vi "cluster2array_for_overlay.vi"(11 "side of clusters":cluster{"Array out":dbl[][]}[](array[cluster])) -> (0 "Left side points":cluster{"X":i32, "Y":i32}[](array[cluster]), 1 "Bottom side points":cluster{"X":i32, "Y":i32}[](array[cluster]), 2 "Right side points":cluster{"X":i32, "Y":i32}[](array[cluster]), 3 "Top side points":cluster{"X":i32, "Y":i32}[](array[cluster]))   [LabVIEW 2017]
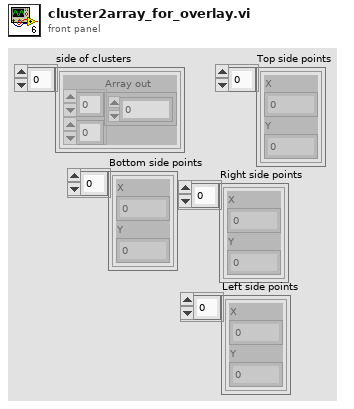
[diagram p1: front panel]
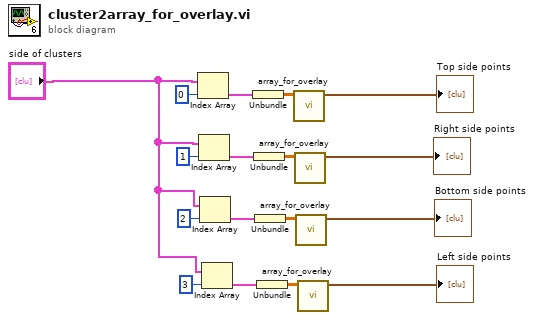
[diagram p0: block diagram]
diagram:
  n1 = Index Array(array="side of clusters", index=0 ("index (page)")) -> (element=w16:cluster{"Array out":dbl[][]})
  n2 = Index Array(array="side of clusters", index=1 ("index (page)")) -> (element=w12:cluster{"Array out":dbl[][]})
  n3 = Index Array(array="side of clusters", index=2 ("index (page)")) -> (element=w9:cluster{"Array out":dbl[][]})
  n4 = Index Array(array="side of clusters", index=3 ("index (page)")) -> (element=w6:cluster{"Array out":dbl[][]})
  n5 = Unbundle(w16) -> ("Array out"=w17:dbl[][])
  n6 = Unbundle(w12) -> ("Array out"=w11:dbl[][])
  n7 = Unbundle(w9) -> ("Array out"=w10:dbl[][])
  n8 = Unbundle(w6) -> ("Array out"=w5:dbl[][])
  n9 = call "array_for_overlay.vi"("Array in"=w17) -> ("Array out"=→"Top side points":cluster{"X":i32, "Y":i32}[])  [unwired: 10 in]
  n10 = call "array_for_overlay.vi"("Array in"=w11) -> ("Array out"=→"Right side points":cluster{"X":i32, "Y":i32}[])  [unwired: 10 in]
  n11 = call "array_for_overlay.vi"("Array in"=w10) -> ("Array out"=→"Bottom side points":cluster{"X":i32, "Y":i32}[])  [unwired: 10 in]
  n12 = call "array_for_overlay.vi"("Array in"=w5) -> ("Array out"=→"Left side points":cluster{"X":i32, "Y":i32}[])  [unwired: 10 in]
